vi "Handle INSERT Error.vi"(8 "error in (no error)":errorcluster, 10 "SQL":string, 11 "Database.PG":refnum<class "LV-Data.PGSQL.lvclass">) -> (0 "error out":errorcluster, 2 "Wrote to DB?":bool, 3 "Database.PG out":refnum<class "LV-Data.PGSQL.lvclass">)   [LabVIEW 2019, in "LV-Data.PGSQL.lvclass"]
uses:
  LV-Data.PGSQL.lvclass
  Push Backup to DB.vi
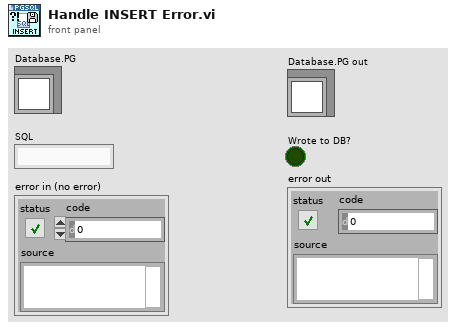
[diagram p1: front panel]
types:
  T1 = enum16{"open", "replace", "create", "open or create", "replace or create", "replace or create with confirmation"}
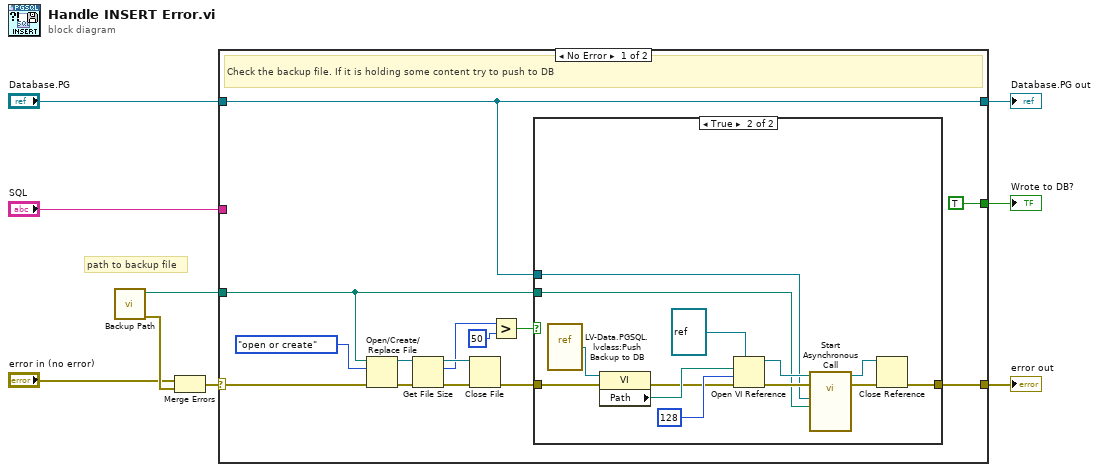
[diagram p0: block diagram]
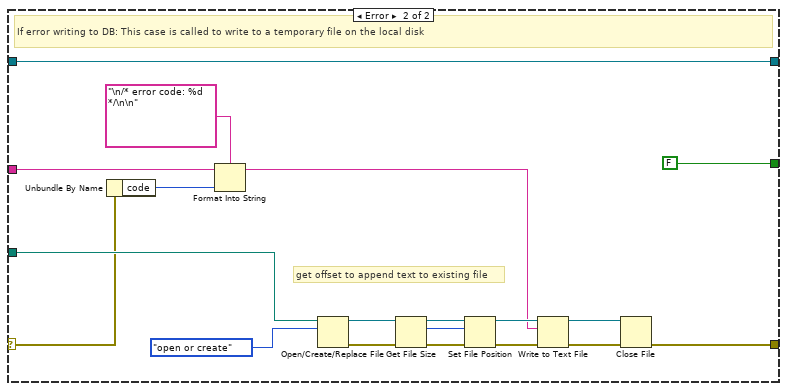
[diagram p3: hidden frame]
diagram:
  # "path to backup file"
  n1 = call "Backup Path.vi"() -> ("error out"=w3:errorcluster, "pg_backup.txt path"=w2:path)  [unwired: 10 in]
  n2 = Merge Errors("error in (no error)", w3) -> (w4:errorcluster)
  n3 = case shown="No Error" w4 {
    selector: w4 -> [w17 w39]
    tunnel: "SQL" -> [_ w56]
    tunnel: [TRUE FALSE] -> w7
    tunnel: "Database.PG" -> [w16 w42]
    tunnel: w2 -> [w12 w43]
    tunnel: [w16 w42] -> w6
    tunnel: [w18 w41] -> w5
    frame No Error {
      # "Check the backup file. If it is holding some content try to push to DB"
      n4 = Open/Create/Replace File(file path (use dialog)=w12, error in=w17, operation (0:open)=T1."open or create") -> (refnum out=w22:refnum<file>, error out=w23:errorcluster)  [unwired: 3 in, 1 out]
      n5 = Get File Size(file=w22, error in=w23) -> (refnum out=w15:refnum<file>, size (in bytes)=w11:i64, 0:w14:errorcluster)
      n6 = Close File(refnum=w15, error in=w14) -> (error out=w13:errorcluster)  [unwired: 1 out]
      n7 = Greater?(x=w11, y=i64 50) -> (0:w20:bool)
      n8 = case shown="True" w20 {
        tunnel: w16 -> [_ w27]
        tunnel: w12 -> [_ w25]
        tunnel: [w24 w26] -> w18
        tunnel: w13 -> [w24 w28]
        frame False {
        }
        frame True {
          n9 = vi-ref "LV-Data.PGSQL.lvclass:Push Backup to DB.vi"() -> (w31:refnum<vi>)
          n10 = property class="VI"(reference=w31, error in=w28) -> (error out=w29:errorcluster, "Path"=w30:path)  [unwired: 1 out]
          n11 = Open VI Reference(type specifier VI Refnum (for type only)=refnum<vi> refnum, vi path=w30, options=128, error in (no error)=w29) -> (vi reference=w36:refnum<vi>, error out=w34:errorcluster)  [unwired: 2 in]
          n12 = call-by-ref "Start Asynchronous Call"(reference=w36, error in=w34, "Path to backup file"=w25, "Data.PG"=w27) -> (reference out=w32:refnum<vi>, error out=w35:errorcluster)  [unwired: 10 in]
          n13 = Close Reference(reference=w32, error in (no error)=w35) -> (error out=w26:errorcluster)
        }
      }
    }
    frame Error {
      # "get offset to append text to existing file"
      # "If error writing to DB: This case is called to write to a temporary file on the local disk"
      n14 = Unbundle By Name(w39) -> ("code"=w44:i32)
      n15 = Format Into String(format string="\n/* error code: %d */\n\n", initial string=w56, w44) -> (resulting string=w50:string)  [unwired: 1 in, 1 out]
      n16 = Open/Create/Replace File(file path (use dialog)=w43, operation (0:open)=T1."open or create") -> (refnum out=w46:refnum<file>, error out=w45:errorcluster)  [unwired: 4 in, 1 out]
      n17 = Get File Size(file=w46, error in=w45) -> (refnum out=w53:refnum<file>, size (in bytes)=w54:i64, 0:w55:errorcluster)
      n18 = Set File Position(offset (in bytes) (0)=w54, refnum=w53, error in=w55) -> (refnum out=w51:refnum<file>, error out=w52:errorcluster)  [unwired: 1 in]
      n19 = Write to Text File(file (use dialog)=w51, text=w50, error in=w52) -> (refnum out=w48:refnum<file>, error out=w49:errorcluster)  [unwired: 1 in, 1 out]
      n20 = Close File(refnum=w48, error in=w49) -> (error out=w41:errorcluster)  [unwired: 1 out]
    }
  }
  "Wrote to DB?" <- w7
  "Database.PG out" <- w6
  "error out" <- w5
